vi "Set Parent.vi"(8 "Error In":errorcluster, 10 "Parent":refnum<class "OD Entry.lvclass">, 11 "reference in":refnum<class "OD Sub-Entry.lvclass">) -> (0 "Error Out":errorcluster, 3 "reference out":refnum<class "OD Sub-Entry.lvclass">)   [LabVIEW 2024, in "Electronic Datasheet.lvlib" / "OD Sub-Entry.lvclass"]
uses:
  OD Sub-Entry.lvclass
  OD Entry/OD Entry.lvclass
  OD Sub-Entry.lvclass/OD Sub-Entry.ctl
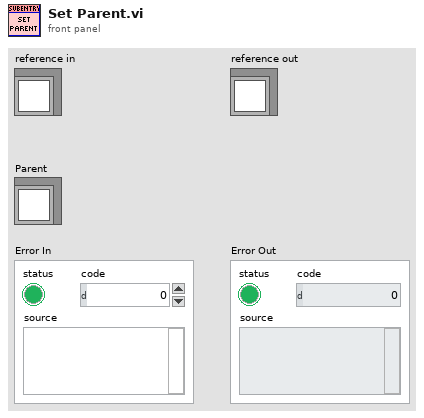
[diagram p1: front panel]
types:
  T1 = typedef "Electronic Datasheet.lvlib/OD Sub-Entry.lvclass/ObjectAttributes.ctl" = cluster{"Parent":refnum<class "OD Entry.lvclass">}
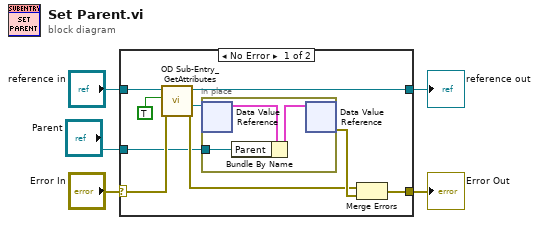
[diagram p0: block diagram]
diagram:
  n1 = case shown="No Error" "Error In" {
    selector: "Error In" -> [w14 w19]
    tunnel: [w11 w19] -> w4
    tunnel: [w9 w18] -> w2
    tunnel: "reference in" -> [w10 w18]
    tunnel: "Parent" -> [w6 _]
    frame No Error {
      n2 = call "OD Sub-Entry_GetAttributes.vi"("Error In"=w14, "OnlyGetDvrReference(False)"=TRUE, "reference in"=w10) -> ("Error Out"=w12:errorcluster, "DataRef"=w7:refnum<data-value>, "reference out"=w9:refnum<class "OD Sub-Entry.lvclass">)  [unwired: 5 in, 1 out]
      n3 = in-place {
        in-place-border: w6 -> [w17]
        n4 = in-place-dvr #1(w7) -> (w16:T1)  [unwired: 1 out]
        n5 = Bundle By Name(cluster=w16, "Parent"=w17) -> (w15:T1)
        n6 = in-place-dvr #1(w15) -> (w13:errorcluster)  [unwired: 1 out]
      }
      n7 = Merge Errors(w12, w13) -> (w11:errorcluster)
    }
    frame Error {
    }
  }
  "Error Out" <- w4
  "reference out" <- w2
